vi "GUI_optionsUpdate.vi"(0 "reference":refnum<class "OSA.lvclass">, 5 "error in (no error)":errorcluster, 6 "ctrl refs":T1) -> (14 "duplicate reference":refnum<class "OSA.lvclass">, 19 "error out":errorcluster)   [LabVIEW 2010, in "OSA.lvclass"]
doc: "Reads the contents of a <B>Thorlabs_OSA_64</B> object.\n\n[GOOP 1.0]"
uses:
  OSA.lvclass
  ctrlRefs.ctl
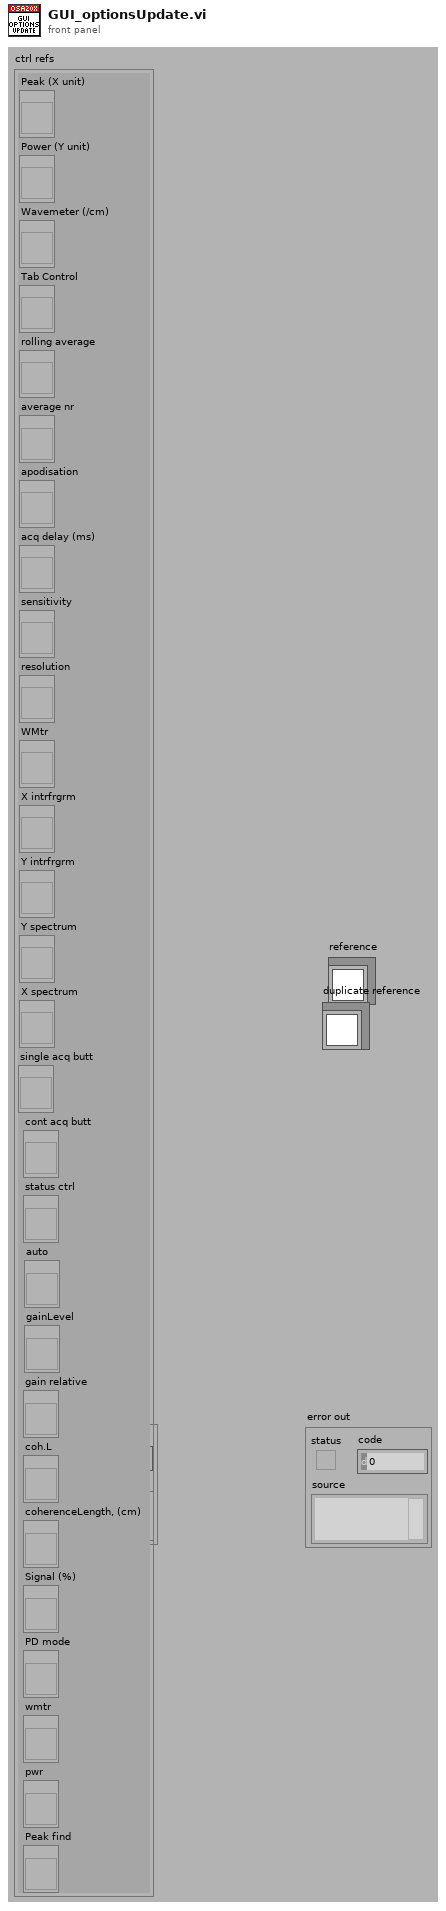
[diagram p1: front panel]
types:
  T1 = typedef "OSA.lvclass/ctrlRefs.ctl" = cluster{"Peak (X unit)":refnum<vi>, "Power (Y unit)":refnum<vi>, "Wavemeter (/cm)":refnum<vi>, "Tab Control":refnum<vi>, "rolling average":refnum<vi>, "average nr":refnum<vi>, "apodisation":refnum<vi>, "acq delay (ms)":refnum<vi>, "sensitivity":refnum<vi>, "resolution":refnum<vi>, "WMtr":refnum<vi>, "X intrfrgrm":refnum<vi>, "Y intrfrgrm":refnum<vi>, "Y spectrum":refnum<vi>, "X spectrum":refnum<vi>, "single acq butt":refnum<vi>, "cont acq butt":refnum<vi>, "status ctrl":refnum<vi>, "auto":refnum<vi>, "gainLevel":refnum<vi>, "gain relative":refnum<vi>, "coh.L":refnum<vi>, "coherenceLength, (cm)":refnum<vi>, "Signal (%)":refnum<vi>, "PD mode":refnum<vi>, "wmtr":refnum<vi>, "pwr":refnum<vi>, "Peak find":refnum<vi>}
  T2 = typedef "OSA.lvclass/ObjectAttributes.ctl" = cluster{"Stop":bool, "dataType":T3, "spectrometerIdx":u16, "buffer size interferogram":i32, "interferogram":cluster{"new":bool, "plot_x_ min":sgl, "plot_x_max":sgl, "plot_y_min":sgl, "plot_y_max":sgl, "Graph Intrfrgrm":T4, "timeStamp":u32, "signal (%)":dbl, "traces":cluster{"idx":u32, "broadBand":bool, "monoChromatic":bool, "peakToPeakSignal":dbl, "peakToPeakPos":dbl}[], "traces idx last":i32}, "spectrum":cluster{"new":bool, "plot_x_min":sgl, "plot_x_max":sgl, "plot_unit_x":T5, "plot_unit_y":T6, "plot_y_min":sgl, "plot_y_max":sgl, "Graph Spectrum":T4, "timeStamp":u32, "X_VAL_OPTIONS":enum16{"MIN_MAX", "ARRAY"}, "traces":cluster{"idx":u32}[], "traces idx last":i32}, "Thorlabs_OSA_64.lvclass:queue_action.ctlqueue ref":refnum<queue>, "action":T7, "plot zoom step":dbl, "buffer semaphore":T8, "acq stopped":bool, "dataType active":T3, "temperature (degr C)":sgl, "pressure (hPa)":sgl, "rel humidity (%)":sgl, "settings":cluster{"resolution":T9, "sensitivity":T10, "Average":bool, "average nr":u32, "apodisation":T11, "acq delay (ms)":u32, "airMesure":T12, "wmtr on":bool, "intfgrm_smooth_width":u16, "intfgrm_smooth_nrOfPasses":u16, "intfgrm_smooth":T13, "phaseCorrection":T14, "zeroFill":u8, "spectr_smooth":T13, "spectr_smooth_width":u16, "spectr_smooth_nrOfPasses":u16, "resolution (/cm)":sgl, "REF wavelength, (nm)":dbl, "gain_idx":u16, "gainAuto":bool, "gain_relative":dbl, "PD sensitivity mode":T15, "PD senseMode implemented":bool, "SensorTemperature implemented":bool, "SensorPressure implemented":bool, "SensorHumidity implemented":bool}, "peaks position":sgl[], "peaks width":sgl[], "peaks height":sgl[], "peaks max nr":u32, "peaks latest nr":i32, "peaks new":bool, "power":dbl, "power new":bool, "path":string, "wavelength (WNr)":dbl, "wavelength new":bool, "buffer size spectrum":i32, "status":string, "VI reference":refnum<vi>, "funcPointer":u64, "libraryPointer":u64, "singleAcquisition":bool, "coherenceLength (cm)":dbl, "coherenceLength new":bool, "spectrometer model":string, "spectrometer serial nr":string, "peaks thld left":sgl[], "peaks thld right":sgl[], "coherenceLength error (cm)":dbl, "ADC bits":u16, "peaks position centroid":sgl[], "peaks height centroid":sgl[], "OSA series":T16, "channel index":u16, "channel index stiched":u16, "spectrum channel type":T17}
  T3 = typedef "OSA.lvclass/acq_dataType.ctl" = enum16{"none", "interferogram", "spectrum"}
  T4 = typedef "OSA.lvclass/graph_intensity.ctl" = refnum<vi>
  T5 = typedef "OSA.lvclass/spectrum_x_unit.ctl" = enum16{"wavenr/cm", "THz", "eV", "nm_air", "nm_vac"}
  T6 = typedef "OSA.lvclass/y_unit.ctl" = enum16{"ADC counts", "dBm pwr absolute", "dBm pwr density", "mW pwr absolute", "mW pwr density"}
  T7 = typedef "OSA.lvclass/queue_action.ctl" = enum16{"none", "stop", "GUI_plotInterferogram", "GUI_plotSpectrum", "GUI_plotInterferogramRescale", "GUI_plotSpectrumRescale", "GUI_plotInterferogramReset", "GUI_plotSpectrumReset", "GUI_plotInterferogramAutoScaleY", "GUI_plotSpectrumAutoScaleY", "GUI_plotInterferogramZoomOut", "GUI_plotSpectrumZoomOut", "GUI_plotInterferogramPane", "GUI_plotSpectrumPane", "GUI_plotInterferogramZoomMouse", "GUI_plotSpectrumZoomMouse", "ENVIRONMENT temperature", "ENVIRONMENT pressure", "MODE_resolution set", "MODE_resolution get", "MODE_sensitivity set", "MODE_sensitivity get", "MODE_PDTemperature set", "MODE_PDTemperature get", "REBOOT/RESET firmware", "ACQASYNC_acquireSingleSpectrum", "ACQASYNC_continuous start", "ACQASYNC_continuous stop\n", "ACQASYNC_get last interferogram", "ACQASYNC_get last spectrum", "ACQASYNC_get last waveNr", "ACQOPT_interferogram smoothing set", "ACQOPT_interferogram smoothing get", "ACQOPT_spectrum smoothing set", "ACQOPT_spectrum smoothing get", "ACQOPT_apodisation type set", "ACQOPT_apodisation type get", "ACQOPT_phase correction type set", "ACQOPT_phase correction type get", "ACQOPT_acqIntervall_set", "ACQOPT_acqIntervall_get", "ACQOPT_average spectrum set", "ACQOPT_average spectrum get", "ACQOPT_rolling average set", "ACQOPT_rolling average get", "ACQOPT_zero fill factor set", "ACQOPT_zero fill factor get", "ACQOPT_cycle counting set", "ACQOPT_cycle counting get", "ACQOPT_air measure option set", "ACQOPT_air measure option get", "ACQOPT_gainLevel auto get", "ACQOPT_gainLevel auto set", "ACQOPT_gainLevel get", "ACQOPT_gainLevel set", "ACQOPT_getAll", "INSTRUMENT_PROPERTY_range_WaveNr_min", "INSTRUMENT_PROPERTY_range_WaveNr_max", "INSTRUMENT_PROPERTY_reference_wavelength_cm^-1", "INSTRUMENT_PROPERTY_samplesPerRefPeriod", "INSTRUMENT_PROPERTY_resolution_waveNrPercm", "INSTRUMENT_PROPERTY_availableGainLevels", "INSTRUMENT_PROPERTY_status", "CONVERT", "ANALYSE_POWER", "ANALYSE_PEAKS", "ANALYSE_WAVELENGTH", "ANALYSE_SPECTRUM", "ANALYSE_INTERFEROGRAM", "ANALYSE_COHERENCE_LENGTH", "MATH", "MATH_power", "MATH_peaks", "FILE", "miscellaneous"}
  T8 = typedef "Semaphore RefNum" = refnum<k1>
  T9 = typedef "OSA.lvclass/resolution.ctl" = enum16{"low", "high"}
  T10 = typedef "OSA.lvclass/sensitivityMode.ctl" = enum16{"low", "low medium", "high medium", "high"}
  T11 = typedef "OSA.lvclass/apodisation.ctl" = enum16{"NONE", "NORTON_BEER_WEAK", "NORTON_BEER_MEDIUM", "NORTON_BEER_STRONG", "TRIANGULAR", "COSINE", "HANN", "HAMMING", "BLACKMANHARRIS3", "BLACKMANHARRIS4", "GAUSSIAN"}
  T12 = typedef "OSA.lvclass/airMeasure.ctl" = enum16{"TEMPERATURE", "PRESSURE"}
  T13 = typedef "OSA.lvclass/smoothing.ctl" = enum16{"NONE", "BINOMIAL", "SAVITSKY_GOLAY", "FOURIER", "MOVING_AVERAGE", "GAUSSIAN"}
  T14 = typedef "OSA.lvclass/phaseCorrection.ctl" = enum16{"NONE", "MERTZ", "FORMAN", "MERTZ_FILE", "FORMAN_FILE", "FUTURE COMP."}
  T15 = typedef "OSA.lvclass/PDTemperatureMode.ctl" = enum16{"cool: better sensitivity/noise floor", "warm: extended wl range"}
  T16 = typedef "OSA.lvclass/OSA_series.ctl" = enum16{"OSA200", "OSA300", "UNKNOWN"}
  T17 = typedef "OSA.lvclass/channelType_spectrum.ctl" = enum16{"SINGLE CHANNEL", "STICHED"}
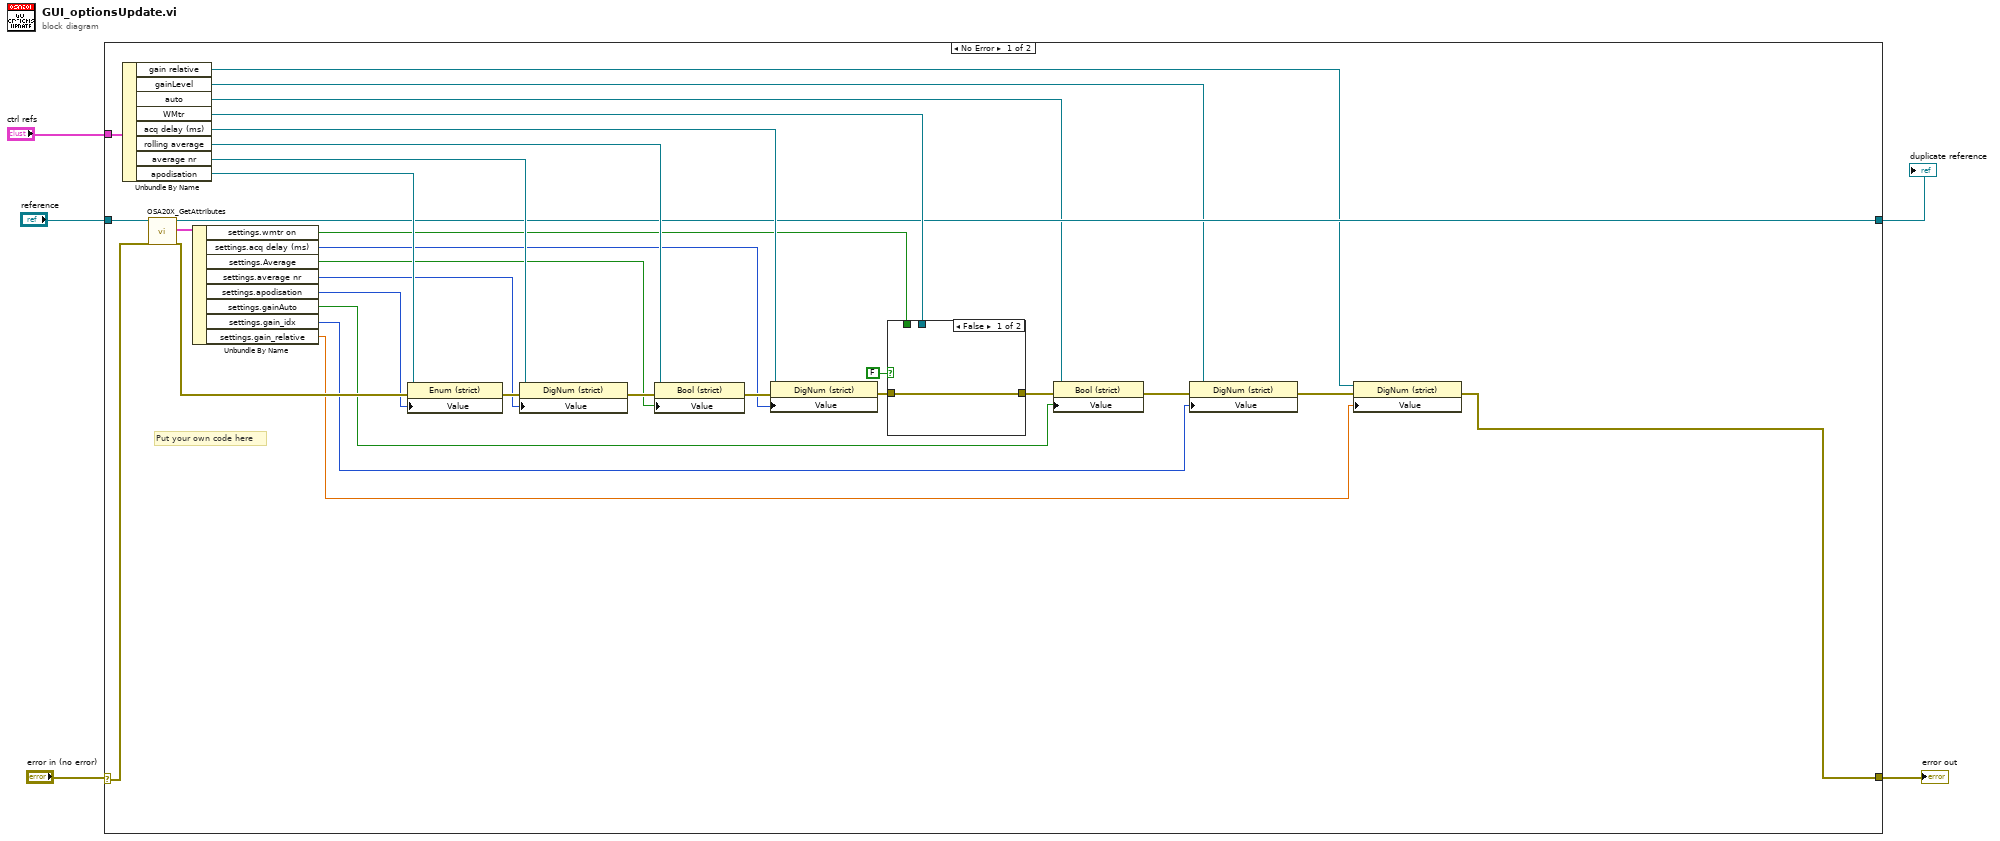
[diagram p0: block diagram]
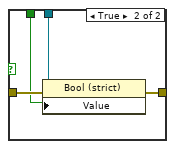
[diagram p2: hidden frame]
diagram:
  n1 = case shown="No Error" "error in (no error)" {
    selector: "error in (no error)" -> [w25 w43]
    tunnel: [w8 w43] -> w5
    tunnel: "ctrl refs" -> [w33 _]
    tunnel: "reference" -> [w26 w42]
    tunnel: [w23 w42] -> w1
    frame No Error {
      # "Put your own code here"
      n2 = Unbundle By Name(w33) -> ("gain relative"=w10:refnum<vi>, "gainLevel"=w16:refnum<vi>, "auto"=w17:refnum<vi>, "WMtr"=w27:refnum<vi>, "acq delay (ms)"=w32:refnum<vi>, "rolling average"=w31:refnum<vi>, "average nr"=w30:refnum<vi>, "apodisation"=w29:refnum<vi>)
      n3 = call "OSA20X_GetAttributes.vi"("reference in"=w26, "error in (no error)"=w25) -> ("reference out"=w23:refnum<class "OSA.lvclass">, "Data"=w7:T2, "error out"=w24:errorcluster)  [unwired: 14 in, 1 out]
      n4 = Unbundle By Name(w7) -> ("settings.wmtr on"=w18:bool, "settings.acq delay (ms)"=w20:u32, "settings.Average"=w19:bool, "settings.average nr"=w21:u32, "settings.apodisation"=w22:T11, "settings.gainAuto"=w13:bool, "settings.gain_idx"=w12:u16, "settings.gain_relative"=w9:dbl)
      n5 = property class="Enum (strict)"(reference=w29, error in=w24, "Value"=w22) -> (error out=w36:errorcluster)  [unwired: 1 out]
      n6 = property class="DigNum (strict)"(reference=w30, error in=w36, "Value"=w21) -> (error out=w35:errorcluster)  [unwired: 1 out]
      n7 = property class="Bool (strict)"(reference=w31, error in=w35, "Value"=w19) -> (error out=w34:errorcluster)  [unwired: 1 out]
      n8 = property class="DigNum (strict)"(reference=w32, error in=w34, "Value"=w20) -> (error out=w28:errorcluster)  [unwired: 1 out]
      n9 = case shown="False" FALSE {
        tunnel: w28 -> [w37 w41]
        tunnel: w27 -> [_ w40]
        tunnel: w18 -> [_ w39]
        tunnel: [w37 w38] -> w15
        frame False {
        }
        frame True {
          n10 = property class="Bool (strict)"(reference=w40, error in=w41, "Value"=w39) -> (error out=w38:errorcluster)  [unwired: 1 out]
        }
      }
      n11 = property class="Bool (strict)"(reference=w17, error in=w15, "Value"=w13) -> (error out=w14:errorcluster)  [unwired: 1 out]
      n12 = property class="DigNum (strict)"(reference=w16, error in=w14, "Value"=w12) -> (error out=w11:errorcluster)  [unwired: 1 out]
      n13 = property class="DigNum (strict)"(reference=w10, error in=w11, "Value"=w9) -> (error out=w8:errorcluster)  [unwired: 1 out]
    }
    frame Error {
      # "Error"
    }
  }
  "error out" <- w5
  "duplicate reference" <- w1
